vi "Init Device.vi"(8 "error in (no error)":errorcluster, 11 "Uniblitz Shutter in":refnum<class "Uniblitz Shutter.lvclass">) -> (0 "error out":errorcluster, 3 "Uniblitz Shutter out":refnum<class "Uniblitz Shutter.lvclass">)   [LabVIEW 2018, in "Uniblitz Shutter.lvlib" / "Uniblitz Shutter.lvclass"]
uses:
  Uniblitz Shutter.lvclass
  Uniblitz Shutter.lvclass/Uniblitz Shutter.ctl
  Resources/Type Defs/Excitation.ctl
  <vilib>/DAQmx/write.llb/DAQmx Write (Digital Bool 1Line 1Point).vi
  <vilib>/DAQmx/create/channels.llb/DAQmx Create Channel (DO-Digital Output).vi
  <vilib>/DAQmx/miscellaneous.llb/DAQmx Fill In Error Info.vi
  Device/Device.lvclass
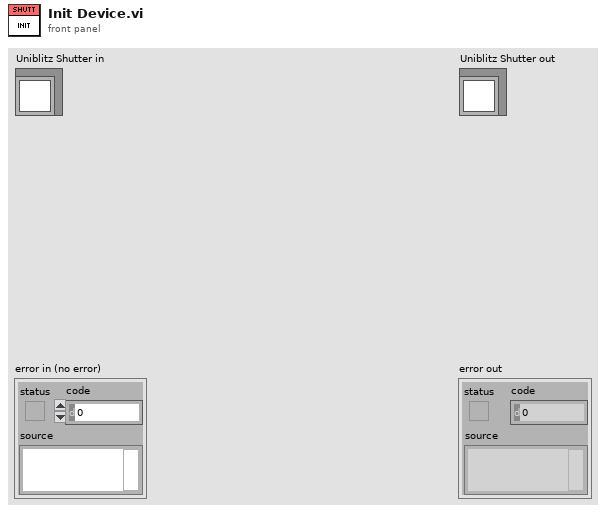
[diagram p1: front panel]
types:
  T1 = typedef "Excitation.ctl" = enum16{"Cy2 (473 nm)", "Cy3 (532 nm)", "Cy5 (639 nm)", "Cy7 (730 nm)", "Cy2/Cy3", "Cy3/Cy5", "Cy3/Cy7", "Cy5/Cy7"}
  T2 = cluster{"Excitation":T1, "DAQmx Channel":refnum<k21>, "Open?":bool}
  T3 = typedef "Shutter Configuration.ctl" = cluster{"IO Line":tag, "Name":string, "Wavelength":u16}
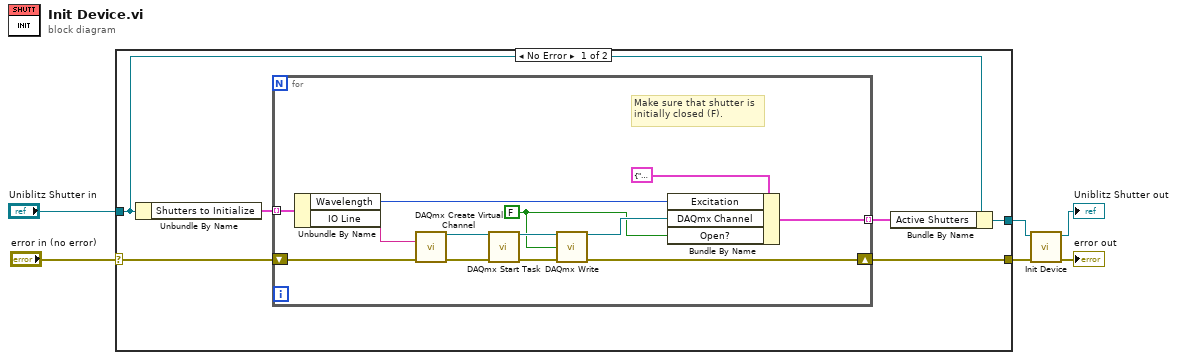
[diagram p0: block diagram]
diagram:
  n1 = case shown="No Error" "error in (no error)" {
    selector: "error in (no error)" -> [w8 w26]
    tunnel: "Uniblitz Shutter in" -> [w11 w27]
    tunnel: [w10 w27] -> w3
    tunnel: [w9 w26] -> w2
    frame No Error {
      n2 = Unbundle By Name(w11) -> ("Shutters to Initialize"=w12:T3[])
      n3 = for {
        tunnel: w12 -> [w16] mode=indexing
        tunnel: [w25] -> w7 mode=indexing
        shift-right: [w17] -> w9
        shift-left: w8 -> [w24]
        w19 = FALSE ("Open?")
        # "Make sure that shutter is\ninitially closed (F)."
        n4 = Unbundle By Name(w16) -> ("Wavelength"=w15:u16, "IO Line"=w14:tag)
        n5 = call-poly <vilib>:"DAQmx Create Virtual Channel.vi"("lines"=w14, "error in"=w24) -> ("task out"=w23:refnum<k21>, "error out"=w22:errorcluster)  [unwired: 12 in]
        n6 = call <vilib>:"DAQmx Start Task.vi"("task/channels in"=w23, "error in"=w22) -> ("task out"=w21:refnum<k21>, "error out"=w18:errorcluster)  [unwired: 12 in]
        n7 = call-poly <vilib>:"DAQmx Write.vi"("task/channels in"=w21, "data"=w19, "error in"=w18) -> ("task out"=w20:refnum<k21>, "error out"=w17:errorcluster)  [unwired: 10 in, 1 out]
        n8 = Bundle By Name(cluster=T2 {"Excitation"=enum."Cy2 (473 nm)", "DAQmx Channel"="", "Open?"=FALSE} ("Properties"), "Excitation"=w15, "DAQmx Channel"=w20, "Open?"=w19) -> (w25:T2)
      }
      n9 = Bundle By Name(cluster=w11, "Active Shutters"=w7) -> (w10:refnum<class "Uniblitz Shutter.lvclass">)
    }
    frame Error {
    }
  }
  n10 = call-parent "Init Device.vi"("error in (no error)"=w2, "Device in"=w3) -> ("error out"=→"error out":errorcluster, "Device out"=→"Uniblitz Shutter out":refnum<class "Uniblitz Shutter.lvclass">)  [unwired: 8 in]
